vi "Memory.Pointer.Get Allocated.vi"(11 "Pointer in":refnum<class "Memory.Pointer.lvclass">) -> (2 "allocated":bool, 3 "Pointer out":refnum<class "Memory.Pointer.lvclass">)   [LabVIEW 2016, in "Memory Manager.lvlib" / "Memory.Pointer.lvclass"]
uses:
  Memory.Pointer.lvclass
  Memory.Pointer.lvclass/Memory.Pointer.ctl
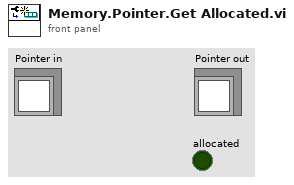
[diagram p1: front panel]
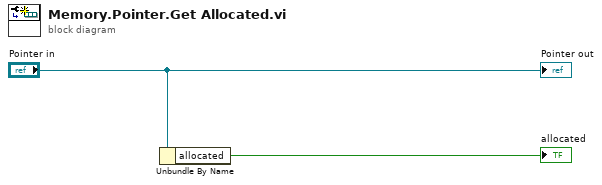
[diagram p0: block diagram]
diagram:
  n1 = Unbundle By Name("Pointer in") -> ("allocated"=→"allocated":bool)
  "Pointer out" <- "Pointer in"
